vi "delete channel none ok.vi"(10 "Sensor Array":T1, 11 "Indexvals in":u32) -> (2 "Sensor Array out":T1, 3 "Indexvals out":u32)   [LabVIEW 2012]
uses:
  DAQ configuration/Sensor array.ctl
  DAQ configuration/channel identifier.ctl
  global scale array.vi
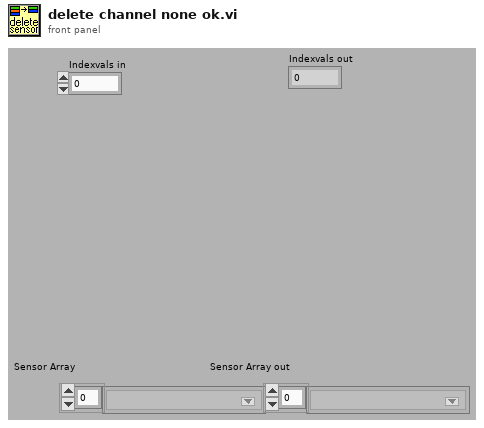
[diagram p1: front panel]
types:
  T1 = typedef "Sensor array.ctl" = T2[]
  T2 = typedef "channel identifier.ctl" = u16
  T3 = typedef "calib array.ctl" = T4[]
  T4 = typedef "conversion.ctl" = cluster{"conversion matrix":sgl[][], "units":string, "name":string, "scale type":T5, "offset (volts)":dbl, "second channel":i8, "correspondence table":T6, "offset (physical units)":dbl, "pH scale":T7, "D.O.":T8}
  T5 = typedef "scale type.ctl" = enum16{"Volts", "Polynomial", "Correspondence Table", "pH", "Dissolved Oxygen", "Quadratic"}
  T6 = typedef "correspondence table.ctl" = cluster{"physical units":dbl, "volts":dbl}[]
  T7 = typedef "pH scale.ctl" = cluster{"Buffers":cluster{"Buffer":dbl, "Calibrated":bool, "V/T":dbl}[], "Temperature":dbl}
  T8 = typedef "DO scale.ctl" = cluster{"Temperature":dbl, "K":dbl, "barometric pressure":dbl}
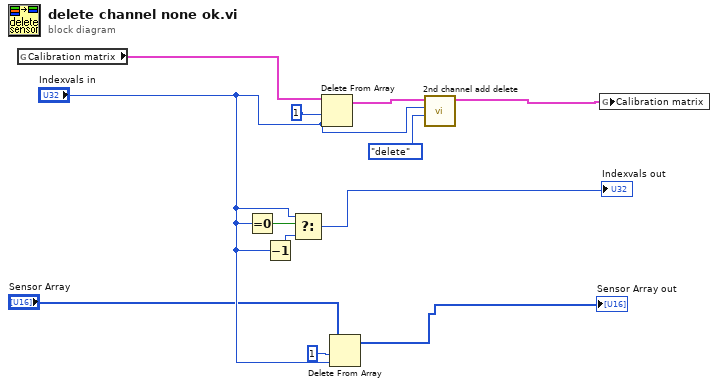
[diagram p0: block diagram]
diagram:
  n1 = global read "global scale array.vi" "Calibration matrix"() -> (w8:T3)
  n2 = Equal To 0?(x="Indexvals in") -> (x = 0?=w2:bool)
  n3 = Decrement(x="Indexvals in") -> (x-1=w1:u32)
  n4 = Select(t="Indexvals in", s=w2, f=w1) -> (s? t:f=→"Indexvals out":u32)
  n5 = Delete From Array(array=w8, length=1 ("Length"), index="Indexvals in") -> (array with subset deleted=w4:T3)  [unwired: 1 out]
  n6 = Delete From Array(array="Sensor Array", length=1 ("Length"), index="Indexvals in") -> (array with subset deleted=→"Sensor Array out":T1)  [unwired: 1 out]
  n7 = call "2nd channel add delete.vi"("action"=enum16{"delete", "insert"}."delete", "Index"="Indexvals in", "Calibration array"=w4) -> ("Calibration array out"=w7:T3)  [unwired: 8 in]
  n8 = global write "global scale array.vi" "Calibration matrix"(w7) -> ()
